vi "Connect Channel Command.vi"(8 "error in":errorcluster, 10 "Channel Connection Data":T1 {"Connection Data" format="%x"}, 11 "ChanMngOOB_Rx in":refnum<class "ChanMngOOB_Rx.lvclass">) -> (0 "error out":errorcluster, 3 "ChanMngOOB_Rx out":refnum<class "ChanMngOOB_Rx.lvclass">)   [LabVIEW 2021, in "ChanMngOOB_Rx.lvclass"]
uses:
  ChanMngOOB_Rx.lvclass
  C:/Program Files/National Instruments/LabVIEW 2021/vi.lib/CIF Foundation/CIF Out of Band Commands/CIFOutOfBand.lvclass
  Typedef/Channel Connection Data.ctl
  <vilib>/CIF Foundation/CIF Out of Band Commands/CIFOutOfBand.lvclass/CIFOutOfBand.ctl
  <vilib>/CIF Foundation/CIF Out of Band Commands/Typedef/OOB Container.ctl
  Typedef/OOB ChnMng Commands.ctl
  Typedef/Template Payload.ctl
  Typedef/Channel Fault Data.ctl
  Typedef/FIFO Publisher.ctl
  <vilib>/CIF Foundation/CIF Channels Core/ChannelCommon/typedef/New FIFO Instance Configuration.ctl
  <vilib>/CIF Foundation/CIF Out of Band Commands/CIFOutOfBand.lvclass
  <vilib>/CIF Foundation/CIF Channels Core/ChannelCommon/ChannelCommon.lvlib
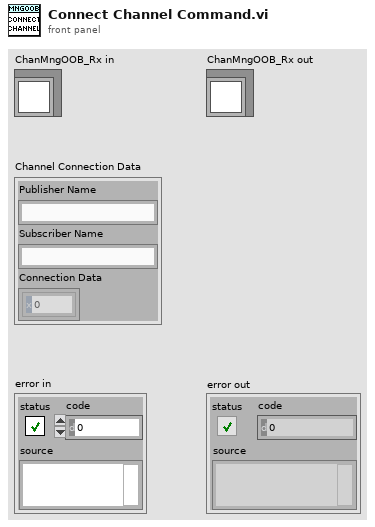
[diagram p1: front panel]
types:
  T1 = typedef "ChanMngOOB_Rx.lvclass/Channel Connection Data.ctl" = cluster{"Publisher Name":string, "Subscriber Name":string, "Connection Data":u8[]}
  T2 = typedef "CIFOutOfBand.lvclass/OOB Container.ctl" = cluster{"Commands (bitwise)":u64, "Payload":variant}
  T3 = typedef "ChanMngOOB_Rx.lvclass/OOB ChnMng Commands.ctl" = enum8{"Connect Channel", "Force Channel", "Add FIFO Pub", "Remove FIFO Pub"}
  T4 = typedef "ChanMngOOB_Rx.lvclass/Template Payload.ctl" = cluster{"Connections":T1[], "Forces":T5[], "FIFO Pub":T6}
  T5 = typedef "ChanMngOOB_Rx.lvclass/Channel Fault Data.ctl" = cluster{"Channel Name":string, "Force Data":u8[], "Force Active":bool}
  T6 = typedef "ChanMngOOB_Rx.lvclass/FIFO Publisher.ctl" = cluster{"Publisher Name":string, "New FIFO Instance Config":T7}
  T7 = typedef "ChannelCommon.lvlib/New FIFO Instance Configuration.ctl" = cluster{"Primary":bool, "Backpressure":bool, "Message/FIFO Override":u32}
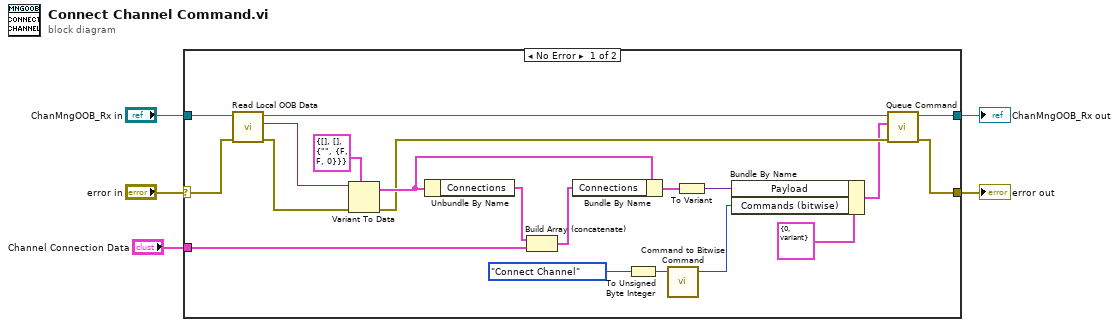
[diagram p0: block diagram]
diagram:
  n1 = case shown="No Error" "error in" {
    selector: "error in" -> [w22 w27]
    tunnel: [w24 w27] -> w4
    tunnel: "ChanMngOOB_Rx in" -> [w23 w26]
    tunnel: [w25 w26] -> w2
    tunnel: "Channel Connection Data" -> [w13 _]
    frame No Error {
      n2 = call <vilib>:"Read Local OOB Data.vi"("error in"=w22, "OOB in"=w23) -> ("error out"=w18:errorcluster, "Local OOB Data"=w21:variant, "OOB out"=w8:refnum<class "ChanMngOOB_Rx.lvclass">)  [unwired: 7 in]
      n3 = Variant To Data(error in=w18, type=T4 {"Connections"=[], "Forces"=[], "FIFO Pub"={"Publisher Name"="", "New FIFO Instance Config"={"Primary"=FALSE, "Backpressure"=FALSE, "Message/FIFO Override"=0}}} ("Template Payload"), Variant=w21) -> (data=w19:T4, error out=w9:errorcluster)
      n4 = Unbundle By Name(w19) -> ("Connections"=w14:T1[])
      n5 = Build Array (concatenate)(w14, w13) -> (w12:T1[])
      n6 = Bundle By Name(cluster=w19, "Connections"=w12) -> (w15:T4)
      n7 = To Unsigned Byte Integer(number=OOB_ChnMng_Commands."Connect Channel" ("OOB Main Commands")) -> (unsigned 8bit integer=w17:u8)
      n8 = call <vilib>:"Command to Bitwise Command.vi"("Command"=w17) -> ("bit command"=w7:u64)  [unwired: 3 in]
      n9 = To Variant(anything=w15) -> (Variant=w10:variant)
      n10 = Bundle By Name(cluster=T2 {"Commands (bitwise)"=0, "Payload"=variant} ("OOB Data"), "Payload"=w10, "Commands (bitwise)"=w7) -> (w6:T2)
      n11 = call <vilib>:"Queue Command.vi"("error in"=w9, "OOB Data"=w6, "OOB in"=w8) -> ("error out"=w24:errorcluster, "OOB out"=w25:refnum<class "ChanMngOOB_Rx.lvclass">)  [unwired: 7 in]
    }
    frame Error {
    }
  }
  "error out" <- w4
  "ChanMngOOB_Rx out" <- w2
